vi "Kalman_smoothing_subVI.vi"(10 "weighting term":dbl, 11 "Signal with  Noise":dynamicdata(waveform)) -> (1 "Raw Data":dbl(slide) scale=-20.0..20.0, 2 "Filtered":dbl(slide) scale=-20.0..20.0, 3 "Compare":cluster{dbl, "data":dbl}(graph))   [LabVIEW 2019]
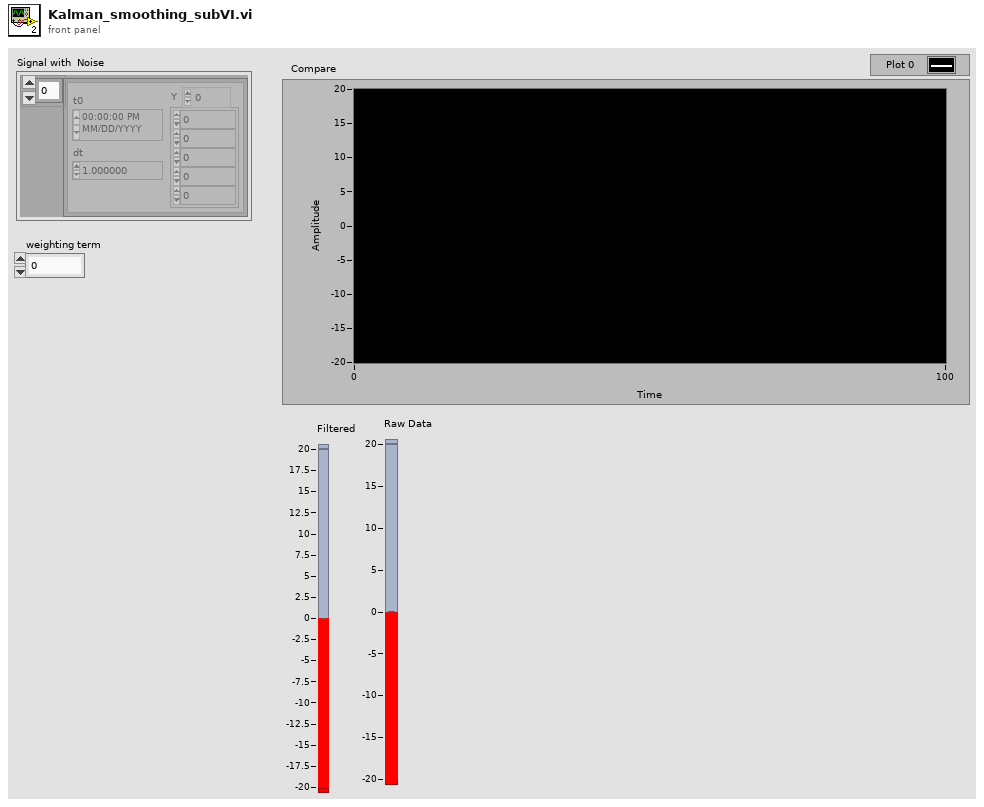
[diagram p1: front panel]
types:
  T1 = cluster{dynamicdata, "Signal with  Noise":dynamicdata}
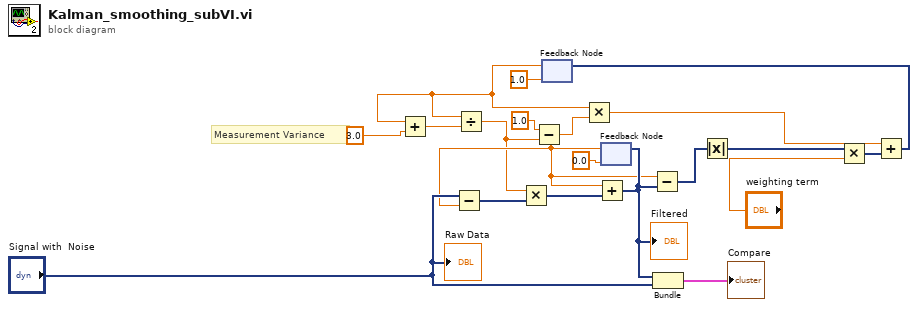
[diagram p0: block diagram]
diagram:
  # "Measurement Variance"
  n1 = feedback #1(1.0) -> (w14:dbl)
  n2 = Add(x=w14, y=3.0) -> (x+y=w2:dbl)
  n3 = Divide(x=w14, y=w2) -> (x/y=w6:dbl)
  n4 = Subtract(x=1.0, y=w6) -> (x-y=w7:dbl)
  n5 = Multiply(x=w14, y=w7) -> (x*y=w8:dbl)
  n6 = feedback #2(0.0) -> (w15:dbl)
  n7 = Subtract(x="Signal with  Noise", y=w15) -> (x-y=w4:dynamicdata)
  n8 = Multiply(x=w6, y=w4) -> (x*y=w3:dynamicdata)
  n9 = Add(x=w15, y=w3) -> (x+y=w19:dynamicdata)
  "Filtered" <- w19
  n10 = feedback-in #2(w19) -> ()
  n11 = Subtract(x=w15, y=w19) -> (x-y=w9:dynamicdata)
  n12 = Bundle(w19, "Signal with  Noise"="Signal with  Noise") -> (→"Compare":T1)  [unwired: 1 in]
  n13 = Absolute Value(x=w9) -> (abs(x)=w10:dynamicdata)
  n14 = Multiply(x=w10, y="weighting term") -> (x*y=w12:dynamicdata)
  n15 = Add(x=w8, y=w12) -> (x+y=w13:dynamicdata)
  n16 = feedback-in #1(w13) -> ()
  "Raw Data" <- "Signal with  Noise"
